vi "Read ProjectName.vi"(11 "Project in":refnum<class "Project.lvclass">) -> (2 "ProjectName":string, 3 "Project out":refnum<class "Project.lvclass">)   [LabVIEW 2021, in "Bananas.lvlib" / "Project.lvclass"]
uses:
  Project.lvclass
  Project.lvclass/Project.ctl
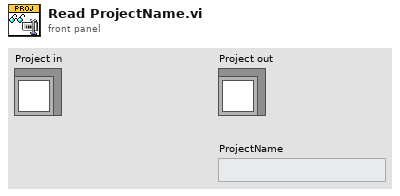
[diagram p1: front panel]
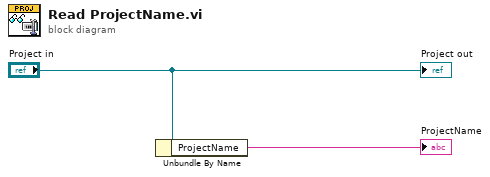
[diagram p0: block diagram]
diagram:
  n1 = Unbundle By Name("Project in") -> ("ProjectName"=→"ProjectName":string)
  "Project out" <- "Project in"
